vi "Preprocess Commands.vi"(11 "Command In":T1={"Name"="", "CPTM.DataType"=variant, "All Control Values Variant"=[], "icon full"={"image type"=0, "image depth"=0, "image"=[], "mask"=[], "colors"=[], "Rectangle"={"left"=0, "top"=0, "right"=0, "bottom"=0}}, "icon scaled"={"image type"=0, "image depth"=0, "image"=[], "mask"=[], "colors"=[], "Rectangle"={"left"=0, "top"=0, "right"=0, "bottom"=0}}, "Path"=path "", "Subsystem Color"=16777216}) -> (3 "Command out":T3)   [LabVIEW 2023]
uses:
  bordeaux-pathinator/Bordeaux/Types/Single Cmd Info.ctl
  <vilib>/picture/picture.llb/imagedata.ctl
panel:
  out "Array":errorcluster[](array[cluster])
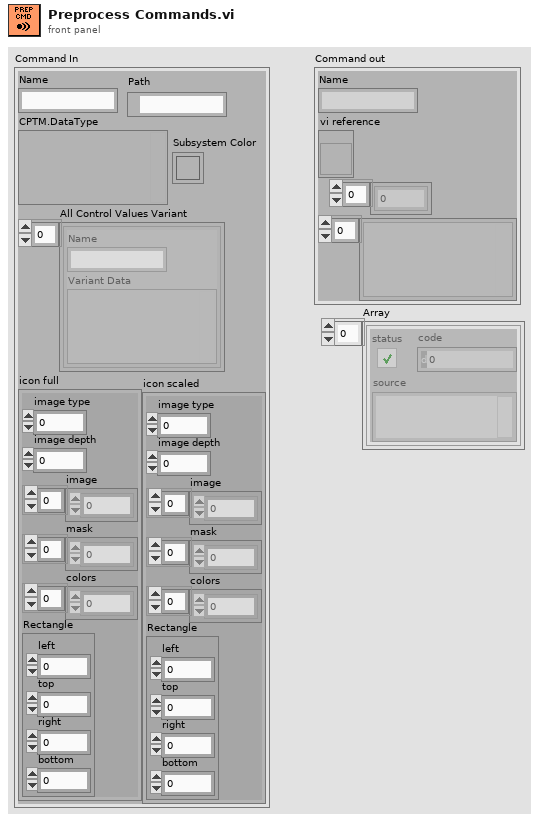
[diagram p1: front panel]
types:
  T1 = typedef "Single Cmd Info.ctl" = cluster{"Name":string, "CPTM.DataType":variant, "All Control Values Variant":cluster{"Name":string, "Variant Data":variant}[], "icon full":T2, "icon scaled":T2, "Path":path, "Subsystem Color":u32}
  T2 = typedef "imagedata.ctl" = cluster{"image type":i32, "image depth":i32, "image":u8[], "mask":u8[], "colors":u32[], "Rectangle":cluster{"left":i16, "top":i16, "right":i16, "bottom":i16}}
  T3 = cluster{"Name":string, "vi reference":refnum<vi>, i32[], variant[]}
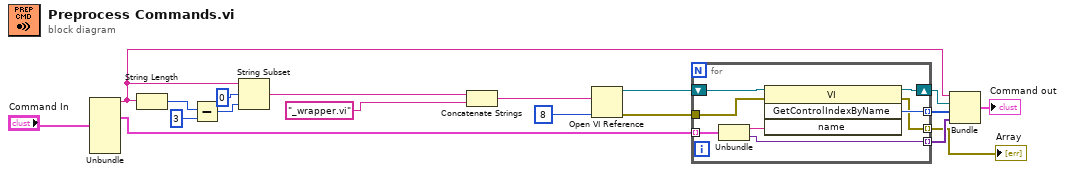
[diagram p0: block diagram]
diagram:
  n1 = Unbundle("Command In") -> ("Name"=w12:string, "All Control Values Variant"=w11:cluster{"Name":string, "Variant Data":variant}[])  [unwired: 5 out]
  n2 = String Length(string=w12) -> (length=w4:i32)
  n3 = Subtract(x=w4, y=3) -> (x-y=w5:i32)
  n4 = String Subset(string=w12, offset (0)=0, length (rest)=w5) -> (substring=w7:string)
  n5 = Concatenate Strings(w7, "_wrapper.vi" ("string")) -> (w9:string)
  n6 = Open VI Reference(vi path=w9, options=8) -> (vi reference=w10:refnum<vi>, error out=w2:errorcluster)  [unwired: 4 in]
  n7 = for {
    tunnel: w11 -> [w24] mode=indexing
    shift-right: [w25] -> w13
    shift-left: w10 -> [w26]
    tunnel: [w22] -> w14 mode=indexing
    tunnel: [w21] -> w15 mode=indexing
    tunnel: w2 -> [w20]
    tunnel: [w19] -> w1 mode=indexing
    n8 = Unbundle(w24) -> ("Name"=w23:string, "Variant Data"=w21:variant)
    n9 = invoke class="VI" method="GetControlIndexByName"(reference=w26, error in=w20, "name"=w23) -> (reference out=w25:refnum<vi>, error out=w19:errorcluster, "GetControlIndexByName"=w22:i32)  [unwired: 1 in, 1 out]
  }
  "Array" <- w1
  n10 = Bundle("Name"=w12, "vi reference"=w13, w14, w15) -> (→"Command out":T3)  [unwired: 1 in]
